vi "Event handler-Dir change.vi"(11 "Old Base Path":path) -> ()   [LabVIEW 2013]
uses:
  Global Variables/gl_UI Ctrl Refs.vi
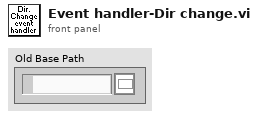
[diagram p1: front panel]
types:
  T1 = typedef "UI ctrl refs cluster.ctl" = cluster{"Top level VI path":path, "Top level VI ref":refnum<vi>, "User menu ref":refnum<k9>, "Sub Panel control":refnum<vi>, "Imaging Param Tab":refnum<vi>, "Occurrence-Start drivers":refnum<k4>, "Occurrence-Speed logging initialised":refnum<k4>, "Occurrence-XYZ stage initialised":refnum<k4>, "Exit button":refnum<vi>, "Status ind":refnum<vi>, "Return to Origin":refnum<vi>, "Speed Logging":refnum<vi>, "Time Lapse":refnum<vi>, "Live Imaging":refnum<vi>, "AOL Z Stack":refnum<vi>, "Motor Z Stack":refnum<vi>, "Funct Acq button":refnum<vi>, "Hard Shutter":refnum<vi>, "Virtual Shutter":refnum<vi>, "Laser Power":refnum<vi>, "AOL Mode":refnum<vi>, "Frame Size":refnum<vi>, "Field of View":refnum<vi>, "Dwell Time":refnum<vi>, "Zoom":refnum<vi>, "AOL Z":refnum<vi>, "Objective":refnum<vi>, "Axis":refnum<vi>, "Paths & Names":refnum<vi>, "Experiment folder path (ind.)":refnum<vi>, "Last State (Ind.)":refnum<vi>, "Laser wavelength ind (nm)":refnum<vi>, "Averages":refnum<vi>, "Angle (degrees)":refnum<vi>, "X centre":refnum<vi>, "Y centre":refnum<vi>, "Plane Mode":refnum<vi>, "# Planes":refnum<vi>, "Z Start":refnum<vi>, "Z Stop":refnum<vi>, "Z Step":refnum<vi>, "PMT 1":refnum<vi>, "PMT 2":refnum<vi>, "Stage XYZ Position":refnum<vi>, "Pockels@Z Start":refnum<vi>, "Pockels@Z Stop":refnum<vi>, "Obtain Z Start":refnum<vi>, "Obtain Z Stop":refnum<vi>, "Live stim.trig.period":refnum<vi>, "Live stim.trig.enable":refnum<vi>, "Funct. Acq. Pockels Modulation":refnum<vi>, "Enable Video Recording":refnum<vi>, "Video Record-Live Imaging":refnum<vi>, "Video Record-Funct acq":refnum<vi>, "AOL Z-stack Chirps Ready (ind)":refnum<vi>, "Center freq ind (nm)":refnum<vi>, "Logging queue (ind)":refnum<vi>, "Back aperture power (ind.)":refnum<vi>, "Power after objective (ind.)":refnum<vi>, "Switch user":refnum<vi>}
  T2 = cluster{"Base Directory":path, "User folder?":bool, "Sub-Folder":string, "Experiment folder custom name":string}
  T3 = typedef "AOL_Globals.ctl" = cluster{"Imaging Protocol":T4, "Number of POI":u16, "Number of Miniscans":u16, "Number of Trials":u16, "Number of Cycles ":u64, "# Averaged Frames":u16, "Laser power (%)":u8, "Pockels":dbl, "Acquisition Length (sec)":dbl, "Fill time (us)":dbl, "POI Dwell time (us)":dbl, "Miniscan Dwell time per pixel (us)":dbl, "PMT 1":dbl, "PMT 2":dbl, "Back Apperture":dbl, "Frame Size":T5, "Center Frequency":dbl, "Field of View":dbl, "DwellTime (us)":dbl, "Wavelength (nm)":dbl, "Zoom":dbl, "AOL Z":dbl, "AOL Mode":T6, "GridXY":dbl, "GridZ":dbl, "TriggerPeriod (sec)":dbl, "Number of Pixels in Miniscan":u16, "Experiment folder path":path, "X centre":dbl, "Y centre":dbl, "Angle (degrees)":dbl, "Plane Mode":T7, "Threshold":u16[], "Regenerate Chirps":bool, "Rectangle ROI length (pixels)":u16, "Rectangle ROI height (pixels)":u16, "AOD fill":u16, "Samples Wait after Trigger":u16, "StartUp Delay":i32, "Slip Cycle":u32, "Add Cycle":bool}
  T4 = typedef "Imaging Protocols enum.ctl" = enum16{"AOL Z-Stack", "Motor Z Stack", "Functional Acquisition", "Single Plane Acquisition", "Volume Acquisition", "Live Imaging", "Live Plane Imaging", "Live Volume Imaging"}
  T5 = typedef "Frame Size.ctl" = u16
  T6 = typedef "AOL modes.ctl" = enum16{"Raster", "Structural", "Pointing", "Mini Scan", "Alignment"}
  T7 = typedef "Plane Mode.ctl" = u16
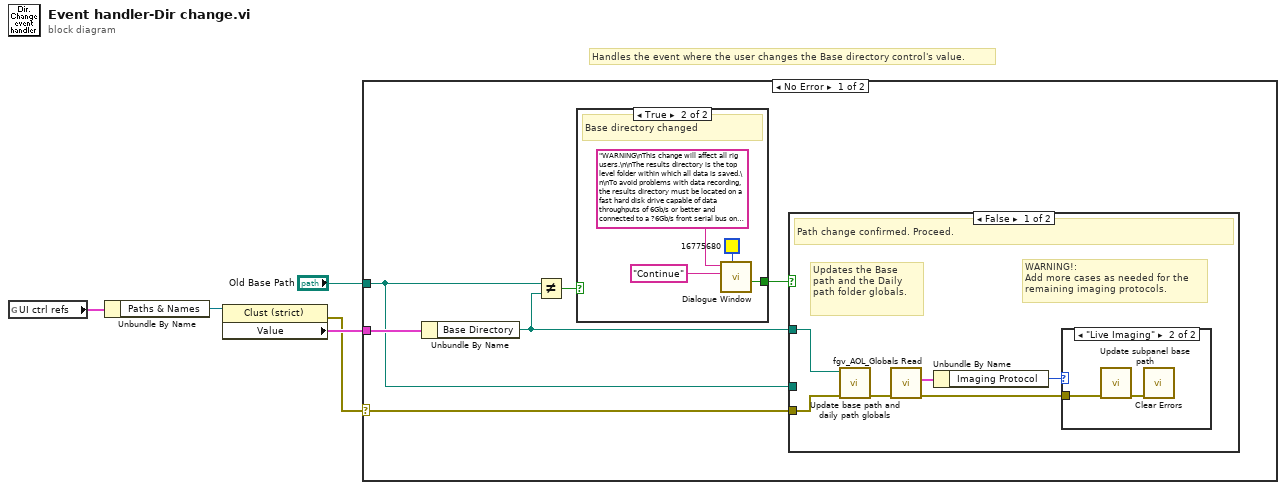
[diagram p0: block diagram]
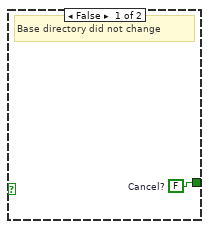
[diagram p2: hidden frame]
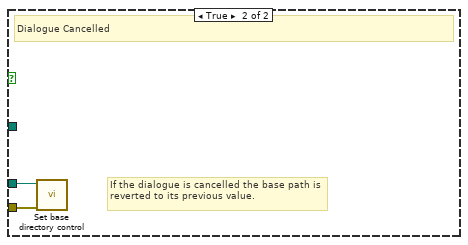
[diagram p4: hidden frame]
diagram:
  # "Handles the event where the user changes the Base directory control's value."
  n1 = global read "gl_UI Ctrl Refs.vi" "UI ctrl refs"() -> (w5:T1)
  n2 = Unbundle By Name(w5) -> ("Paths & Names"=w4:refnum<vi>)
  n3 = property class="Clust (strict)"(reference=w4) -> (error out=w2:errorcluster, "Value"=w3:T2)  [unwired: 1 in, 1 out]
  n4 = case shown="No Error" w2 {
    selector: w2 -> [w10 _]
    tunnel: w3 -> [w11 _]
    tunnel: "Old Base Path" -> [w6 _]
    frame No Error {
      n5 = Unbundle By Name(w11) -> ("Base Directory"=w9:path)
      n6 = Not Equal?(x=w6, y=w9) -> (x != y?=w8:bool)
      n7 = case shown="True" w8 {
        tunnel: [w12 w15] -> w7
        frame False {
          w12 = FALSE  # Cancel?
          # "Base directory did not change"
        }
        frame True {
          # "Base directory changed"
          n8 = call "Dialogue Window.vi"("Colour"=u32 16775680, "Caption-Right button (OK)"="Continue", "Message string"="WARNING\nThis change will affect all rig users.\n\nThe results directory is the top level folder within which all data is saved.\n\nTo avoid problems with data recording, the results directory must be located on a fast hard disk drive capable of data throughputs of 6Gb/s or better and connected to a ?6Gb/s front serial bus on the computer's motherboard.\n\nAre you sure you want to continue?\n") -> ("Cancelled (Left button pressed)"=w15:bool)  [unwired: 6 in, 2 out]
        }
      }
      n9 = case shown="False" w7 {
        tunnel: w10 -> [w19 w25]
        tunnel: w9 -> [w20 _]
        tunnel: w6 -> [_ w26]
        frame False {
          # "Updates the Base path and the Daily path folder globals."
          # "WARNING!:\nAdd more cases as needed for the remaining imaging protocols."
          # "Path change confirmed. Proceed."
          n10 = call "Update base path and daily path globals.vi"("error in"=w19, "Base Directory"=w20) -> ("error out"=w17:errorcluster)  [unwired: 8 in, 1 out]
          n11 = call "fgv_AOL_Globals Read.vi"("error in (no error)"=w17) -> ("error out"=w18:errorcluster, "AOL_Globals"=w21:T3)  [unwired: 8 in, 1 out]
          n12 = Unbundle By Name(w21) -> ("Imaging Protocol"=w22:T4)
          n13 = case shown="\"Live Imaging\"" w22 {
            tunnel: w18 -> [_ w23]
            frame Default {
            }
            frame "Live Imaging" {
              n14 = call "Update subpanel base path.vi"("error in (no error)"=w23) -> ("error out"=w24:errorcluster)  [unwired: 10 in]
              n15 = call <vilib>:"Clear Errors.vi"("error in (no error)"=w24) -> ()  [unwired: 6 in, 1 out]
            }
          }
        }
        frame True {
          # "If the dialogue is cancelled the base path is reverted to its previous value."
          # "Dialogue Cancelled"
          n16 = call "Set base directory control.vi"("error in (no error)"=w25, "Base path"=w26) -> ()  [unwired: 9 in, 1 out]
        }
      }
    }
    frame Error {
    }
  }
